vi "Associate Instruments to Paths.vi"(0 "Scalar SG Path Group in":refnum<class "SG SC2250 Path Group.lvclass">, 5 "TSM Context":T1, 11 "error in (no error)":errorcluster) -> (4 "Scalar SG Path Group out":refnum<class "SG SC2250 Path Group.lvclass">, 15 "error out":errorcluster)   [LabVIEW 2023, in "RFFixtureCharact.RFPM.lvlib" / "SG SC2250 Path Group.lvclass"]
uses:
  SG SC2250 Path Group.lvclass
  C:/srd-semi-rfcal-software/AuxTools/STSRFFixtureCharactUtility/Source/Code Modules/Common/Base Classes/Path Group/Path Group.lvclass
  <vilib>/NI_TestStand_SemiconductorModule/NI_TestStand_Semiconductor_Module.lvlibp/PinMap/General/SemiconductorModuleContext.ctl
  Paths/SG SC2250 Path/SG SC2250 Path.lvclass
  C:/srd-semi-rfcal-software/AuxTools/STSRFFixtureCharactUtility/Source/Code Modules/Fixture/Public/Base Classes/Scalar/SG Abstract Path/SG Abstract Path.lvclass
  C:/srd-semi-rfcal-software/AuxTools/STSRFFixtureCharactUtility/Source/Code Modules/Common/Base Classes/Path/Path.lvclass
  C:/srd-semi-rfcal-software/AuxTools/STSRFFixtureCharactUtility/Source/Code Modules/Fixture/Public/Base Classes/Scalar/Scalar Path/Scalar Path.lvclass
  C:/srd-semi-rfcal-software/AuxTools/STSRFFixtureCharactUtility/Source/Code Modules/Fixture/RFPM/Scalar/Paths/SG Path/SG 18GHz Path.lvclass
  Public/Base Classes/Scalar/SG Abstract Path/SG Abstract Path.lvclass
  <instrlib>/si2250/si2250.llb/si2250 TX Output Path.ctl
  Charact Result Accessor/Scalar/Scalar Charact Result Accessor.lvclass
  C:/srd-semi-rfcal-software/AuxTools/STSRFFixtureCharactUtility/Source/Code Modules/Fixture/RFPM/Charact Result Accessor/Base/Charact Result Accessor.lvclass
  C:/srd-semi-rfcal-software/AuxTools/STSRFFixtureCharactUtility/Source/Code Modules/Common/Result Accessor/Result Accessor.lvclass
  Paths/SG SC2250 Path/SG SC2250 Path.lvclass/SG SC2250 Path.ctl
  Paths/SG SC2250 Path/Properties/Read Cal Tone Source.vi
  Paths/SG SC2250 Path/Properties/Write SC2250 Session.vi
  <vilib>/NI_TestStand_SemiconductorModule/NI_TestStand_Semiconductor_Module.lvlibp/PinMap/RF/RFmx/PinToNIRFmxSession.vi
  <vilib>/NI_TestStand_SemiconductorModule/NI_TestStand_Semiconductor_Module.lvlibp/PinMap/RF/RFPM/PinToNIRFPMSessionsWithPaths.vi
  <vilib>/NI_TestStand_SemiconductorModule/NI_TestStand_Semiconductor_Module.lvlibp/PinMap/RF/RFSG/PinToNIRFSGSession.vi
  Common/Base Classes/Path/Path.lvclass
  Common/Result Accessor/Result Accessor.lvclass
  <vilib>/NI_TestStand_SemiconductorModule/NI_TestStand_Semiconductor_Module.lvlibp
  Common/Base Classes/Path Group/Path Group.lvclass
  Instruments/Power Meter/Power Meter Factory/Power Meter Factory.lvclass
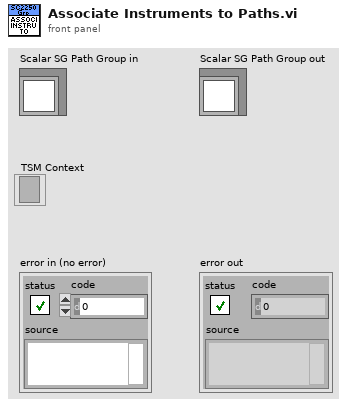
[diagram p1: front panel]
types:
  T1 = typedef "NI_TestStand_Semiconductor_Module.lvlibp/SemiconductorModuleContext.ctl" = refnum<k7>
  T2 = typedef "si2250 TX Output Path.ctl" = i32
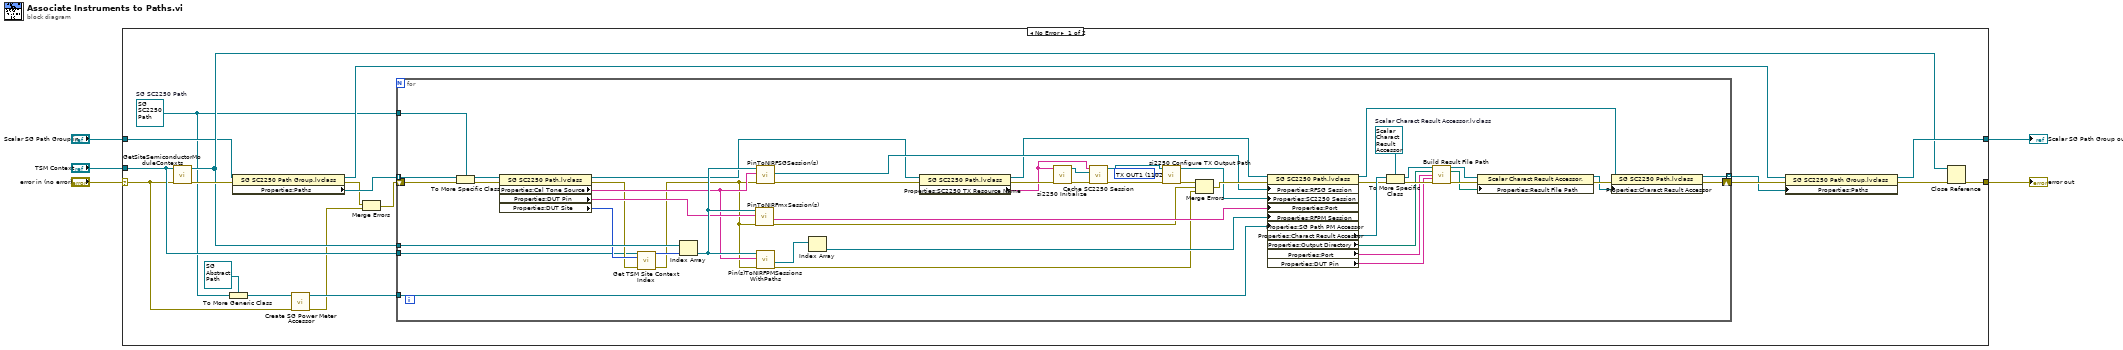
[diagram p0: block diagram]
diagram:
  n1 = case shown="No Error" "error in (no error)" {
    selector: "error in (no error)" -> [w9 w75]
    tunnel: "Scalar SG Path Group in" -> [w16 w76]
    tunnel: [w21 w76] -> w4
    tunnel: "TSM Context" -> [w15 _]
    tunnel: [w18 w75] -> w1
    frame No Error {
      w7 = refnum<class "SG SC2250 Path.lvclass"> refnum  # SG SC2250 Path
      n2 = call <vilib>:"GetSiteSemiconductorModuleContexts.vi"("error in (no error)"=w9, "Semiconductor Module Context"=w15) -> ("error out"=w20:errorcluster, "Site Semiconductor Module Contexts"=w17:T1[])  [unwired: 8 in]
      n3 = To More Generic Class(target class=refnum<class "SG Abstract Path.lvclass"> refnum ("SG Path"), reference=w7) -> (generic class reference=w6:refnum<class "SG Abstract Path.lvclass">)
      n4 = property class="SG SC2250 Path Group.lvclass"(reference=w16, error in=w20) -> (reference out=w22:refnum<class "SG SC2250 Path Group.lvclass">, error out=w12:errorcluster, "Properties:Paths"=w24:refnum<class "Path.lvclass">[])
      n5 = call "Create SG Power Meter Accessor.vi"("SG Path"=w6, "error in"=w9) -> ("SG Path PM Accessor out"=w14:refnum<class "SG Path PM Accessor Base.lvclass">, "error out"=w10:errorcluster)  [unwired: 12 in]
      n6 = Merge Errors(w12, w10) -> (w11:errorcluster)
      n7 = for {
        tunnel: w24 -> [w72] mode=indexing
        shift-right: [w36] -> w23
        shift-left: w11 -> [w59]
        tunnel: [w35] -> w19 mode=indexing
        tunnel: w17 -> [w69]
        tunnel: w15 -> [w50]
        tunnel: w14 -> [w42]
        tunnel: w7 -> [w41]
        w40 = refnum<class "Scalar Charact Result Accessor.lvclass"> refnum  # Scalar Charact Result Accessor.lvclass
        w74 = T2 1102 items=["TX OUT0 Direct"=1100, "TX OUT0 Filter"=1101, "TX OUT1"=1102, "TX OUT2 Internal"=1103] ("Output Path")
        n8 = To More Specific Class(target class=w41, reference=w72, error in=w59) -> (specific class reference=w71:refnum<class "SG SC2250 Path.lvclass">, error out=w58:errorcluster)
        n9 = property class="SG SC2250 Path.lvclass"(reference=w71, error in=w58) -> (reference out=w48:refnum<class "SG SC2250 Path.lvclass">, error out=w52:errorcluster, "Properties:Cal Tone Source"=w54:string, "Properties:DUT Pin"=w55:string, "Properties:DUT Site"=w68:i32)
        n10 = call "Get TSM Site Context Index.vi"("Semiconductor Module Context"=w50, "Site Number"=w68, "error in (no error)"=w52) -> ("index of Site TSM Context"=w53:i32, "error out"=w51:errorcluster)  [unwired: 11 in]
        n11 = Index Array(array=w69, index=w53) -> (element=w64:T1)
        n12 = call-poly <vilib>:"PinToNIRFmxSession(s).vi"("error in (no error)"=w51, "Pin"=w55, "Semiconductor Module Context"=w64) -> ("error out"=w62:errorcluster, "Port"=w63:string)  [unwired: 4 in, 3 out]
        n13 = call-poly <vilib>:"PinToNIRFSGSession(s).vi"("error in (no error)"=w51, "Pin"=w54, "Semiconductor Module Context"=w64) -> ("error out"=w60:errorcluster, "Instrument Session"=w56:refnum<k15>)  [unwired: 4 in, 3 out]
        n14 = call-poly <vilib>:"Pin(s)ToNIRFPMSessionsWithPaths.vi"("error in (no error)"=w51, "Pin"=w54, "Semiconductor Module Context"=w64) -> ("error out"=w61:errorcluster, "Instrument Sessions"=w70:refnum<k15>[])  [unwired: 3 in, 4 out]
        n15 = Index Array(array=w70) -> (element=w67:refnum<k15>)  [unwired: 1 in]
        n16 = property class="SG SC2250 Path.lvclass"(reference=w48, error in=w60) -> (reference out=w47:refnum<class "SG SC2250 Path.lvclass">, error out=w49:errorcluster, "Properties:SC2250 TX Resource Name"=w44:string)
        n17 = call <instrlib>:"si2250 Initialize.vi"("error in"=w49, "resource name"=w44) -> ("error out"=w73:errorcluster, "instrument handle"=w45:refnum<k15>)  [unwired: 8 in]
        n18 = call "Cache SC2250 Session.vi"("Instrument name"=w44, "sc2250 session in"=w45, "error in (no error)"=w73) -> ("sc2250 session out"=w43:refnum<k15>, "error out"=w46:errorcluster)  [unwired: 11 in]
        n19 = call <instrlib>:"si2250 Configure TX Output Path.vi"("error in"=w46, "Output Path"=w74, "instrument handle"=w43) -> ("error out"=w66:errorcluster, "instrument handle out"=w57:refnum<k15>)  [unwired: 7 in]
        n20 = Merge Errors(w66, w62, w61) -> (w65:errorcluster)
        n21 = property class="SG SC2250 Path.lvclass"(reference=w47, error in=w65, "Properties:RFSG Session"=w56, "Properties:SC2250 Session"=w57, "Properties:Port"=w63, "Properties:RFPM Session"=w67, "Properties:SG Path PM Accessor"=w42) -> (reference out=w33:refnum<class "SG SC2250 Path.lvclass">, error out=w34:errorcluster, "Properties:Charact Result Accessor"=w37:refnum<class "Result Accessor.lvclass">, "Properties:Output Directory"=w27:path, "Properties:Port"=w26:string, "Properties:DUT Pin"=w25:string)
        n22 = To More Specific Class(target class=w40, reference=w37, error in=w34) -> (specific class reference=w32:refnum<class "Scalar Charact Result Accessor.lvclass">, error out=w30:errorcluster)
        n23 = call-dynamic "Build Result File Path.vi"("Charact Result Accessor in"=w32, "Output Directory"=w27, "Port 1"=w26, "Port 2"=w25, "error in"=w30) -> ("Charact Result Accessor out"=w31:refnum<class "Scalar Charact Result Accessor.lvclass">, "Result File Path"=w28:path, "error out"=w29:errorcluster)  [unwired: 8 in]
        n24 = property class="Scalar Charact Result Accessor."(reference=w31, error in=w29, "Properties:Result File Path"=w28) -> (reference out=w38:refnum<class "Scalar Charact Result Accessor.lvclass">, error out=w39:errorcluster)
        n25 = property class="SG SC2250 Path.lvclass"(reference=w33, error in=w39, "Properties:Charact Result Accessor"=w38) -> (reference out=w35:refnum<class "SG SC2250 Path.lvclass">, error out=w36:errorcluster)
      }
      n26 = property class="SG SC2250 Path Group.lvclass"(reference=w22, error in=w23, "Properties:Paths"=w19) -> (reference out=w21:refnum<class "SG SC2250 Path Group.lvclass">, error out=w13:errorcluster)
      n27 = Close Reference(reference=w17, error in (no error)=w13) -> (error out=w18:errorcluster)
    }
    frame Error {
    }
  }
  "error out" <- w1
  "Scalar SG Path Group out" <- w4
